vi "Add.vi"(8 "error in (no error)":errorcluster, 9 "parent tag":string, 10 "Destinations in":refnum<class "IB_Destination.lvclass">[](array[class]), 11 "userLabel in":refnum<class "userLabel.lvclass">) -> (0 "error out":errorcluster, 1 "duplicate?":bool, 2 "Destinations out":refnum<class "IB_Destination.lvclass">[](array[class]), 3 "userLabel out":refnum<class "userLabel.lvclass">)   [LabVIEW 2020, in "userLabel.lvclass"]
uses:
  <vilib>/AppBuilder/IB_Classes/Destination/userLabel/userLabel.lvclass
  <vilib>/AppBuilder/IB_Classes/Destination/userLabel/userLabel.lvclass/userLabel.ctl
  <vilib>/AppBuilder/IB_Classes/Destination/IB_Destination.lvclass
  e:/builds/penguin/labview/branches/2020/dev/dist/vi.lib/AppBuilder/IB_Classes/Destination/IB_Destination.lvclass
  e:/builds/penguin/labview/branches/2020/dev/dist/vi.lib/AppBuilder/IB_Classes/Destination/userLabel/userLabel.lvclass
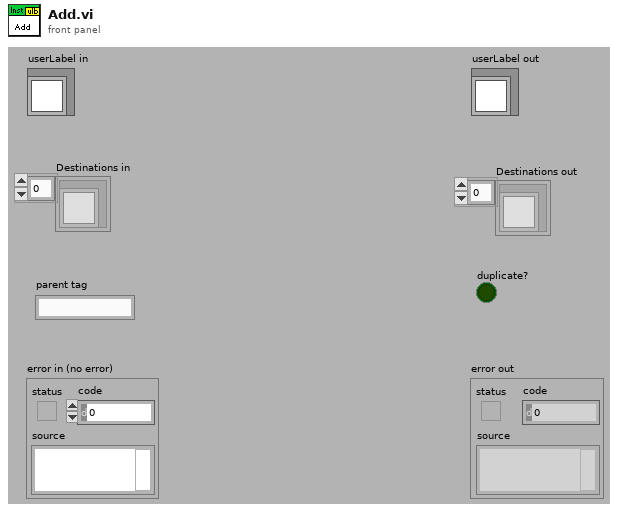
[diagram p1: front panel]
types:
  T1 = typedef "IB_Destination.ctl" = cluster{"name":string, "unlock":bool, "parentTag":string, "destTag":string, "eng_installPath":string}
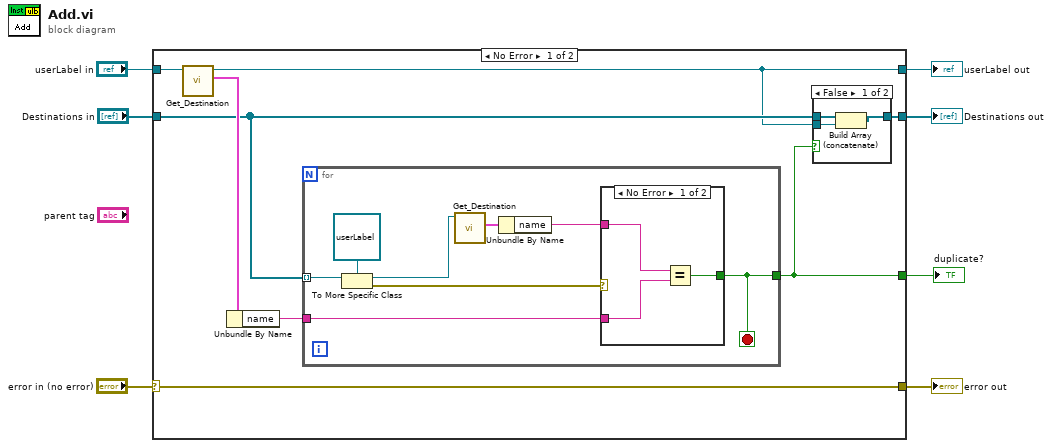
[diagram p0: block diagram]
diagram:
  n1 = case shown="No Error" "error in (no error)" {
    selector: "error in (no error)" -> [w15 w33]
    tunnel: [w15 w33] -> w6
    tunnel: "Destinations in" -> [w11 w31]
    tunnel: "userLabel in" -> [w13 w32]
    tunnel: [w8 _] -> w3
    tunnel: [w9 w32] -> w2
    tunnel: [w10 w31] -> w1
    frame No Error {
      n2 = call <vilib>:"Get_Destination.vi"("IB_Destination in"=w13) -> ("data"=w14:T1, "IB_Destination out"=w9:refnum<class "userLabel.lvclass">)  [unwired: 1 in, 8 out]
      n3 = Unbundle By Name(w14) -> ("name"=w12:string)
      n4 = for {
        tunnel: w11 -> [w27] mode=indexing
        tunnel: w12 -> [w21]
        tunnel: [w20] -> w8
        stop <- w20 stop-if-true
        n5 = To More Specific Class(target class=refnum<class "userLabel.lvclass"> refnum ("userLabel in"), reference=w27) -> (specific class reference=w25:refnum<class "userLabel.lvclass">, error out=w26:errorcluster)  [unwired: 1 in]
        n6 = call <vilib>:"Get_Destination.vi"("IB_Destination in"=w25) -> ("data"=w24:T1)  [unwired: 1 in, 9 out]
        n7 = Unbundle By Name(w24) -> ("name"=w23:string)
        n8 = case shown="No Error" w26 {
          tunnel: w23 -> [w30 _]
          tunnel: w21 -> [w29 _]
          tunnel: [w28 _] -> w20
          frame No Error {
            n9 = Equal?(x=w30, y=w29) -> (x = y?=w28:bool)
          }
          frame Error {
          }
        }
      }
      n10 = case shown="False" w8 {
        tunnel: w11 -> [w18 w19]
        tunnel: [w17 w19] -> w10
        tunnel: w9 -> [w16 _]
        frame False {
          n11 = Build Array (concatenate)(w18, w16) -> (w17:refnum<class "IB_Destination.lvclass">[])
        }
        frame True {
        }
      }
    }
    frame Error {
    }
  }
  "error out" <- w6
  "userLabel out" <- w2
  "Destinations out" <- w1
  "duplicate?" <- w3
